vi "SubVI_RampingDrive_TeleOp.vi"(8 "error in (no error)":errorcluster, 10 "joystick Y Input":dbl) -> (0 "error out":errorcluster, 2 "joystick Y Output":dbl)   [LabVIEW 2017]
uses:
  <vilib>/Rock Robotics/WPI/Solenoid/WPI_SolenoidValue.ctl
  <vilib>/Rock Robotics/WPI/ThirdParty/Phoenix-LabVIEW/Motor Controller/Get/CTRE_Phoenix_MotorController_GetSelectedSensorData.vi
  <vilib>/Rock Robotics/WPI/Solenoid/WPI_SolenoidSetEnum.vi
panel:
  out "joystick Y Output 2":dbl
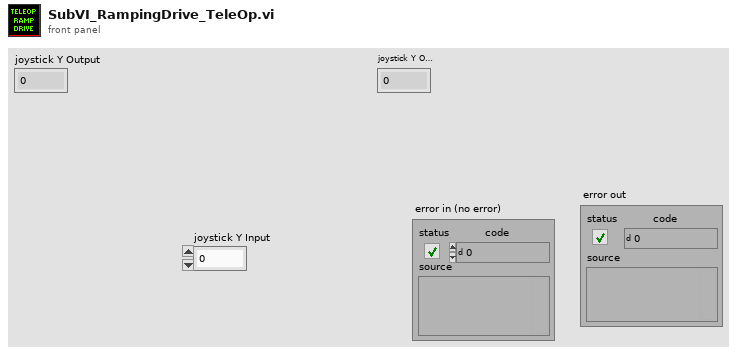
[diagram p1: front panel]
types:
  T1 = typedef "WPI_SolenoidValue.ctl" = enum16{"Off", "On", "Forward", "Reverse"}
  T2 = typedef "WPI_MotorControlDeviceRef.ctl" = cluster{"DeviceStatus":errorcluster, "Type":T3, "PWM":cluster{"PWM Channel":T4, "DeadBand":T5}, "CAN":cluster{"Device Number":u8, "SetOutput VI Ref":variant, "GetOutput VI Ref":variant, "Enable VI Ref":variant, "Disable VI Ref":variant, "Data":variant}, "Invert":bool, "DIO PWM":cluster{"PWM \"Enable\" Channel":T4, "DIOChannel":T6, "PWM Rate":dbl}}
  T3 = typedef "WPI_MotorControlType.ctl" = enum16{"PWM", "CAN", "DIO PWM"}
  T4 = typedef "FPGA_DIOPWMChannel.ctl" = enum8{"PWM 0", "PWM 1", "PWM 2", "PWM 3", "PWM 4", "PWM 5", "PWM 6", "PWM 7", "PWM 8", "PWM 9", "PWM MXP 0", "PWM MXP 1", "PWM MXP 2", "PWM MXP 3", "PWM MXP 4", "PWM MXP 5", "PWM MXP 6", "PWM MXP 7", "PWM MXP 8", "PWM MXP 9", "Invalid"}
  T5 = typedef "WPI_PWMDeadband.ctl" = cluster{"Name":string, "maxPositivePwm":i32, "minPositivePwm":i32, "centerPwm":i32, "maxNegativePwm":i32, "minNegativePwm":i32, "angularRange":u16}
  T6 = typedef "FPGA_DIOChannel.ctl" = enum8{"DIO 0", "DIO 1", "DIO 2", "DIO 3", "DIO 4", "DIO 5", "DIO 6", "DIO 7", "DIO 8", "DIO 9", "DIO MXP 0", "DIO MXP 1", "DIO MXP 2", "DIO MXP 3", "DIO MXP 4", "DIO MXP 5", "DIO MXP 6", "DIO MXP 7", "DIO MXP 8", "DIO MXP 9", "DIO MXP 10", "DIO MXP 11", "DIO MXP 12", "DIO MXP 13", "DIO MXP 14", "DIO MXP 15", "SPI Port CS1", "SPI Port CS2", "SPI Port CS3", "SPI Port MISO", "SPI Port MOSI", "Invalid"}
  T7 = typedef "WPI_SolenoidDevRef.ctl" = cluster{"DevStatus":errorcluster, "Pneumatics Control Module":u8, "Forward Solenoid Channel":T8, "Reverse Solenoid Channel":T8}
  T8 = typedef "WPI_SolenoidChannel.ctl" = enum8{"Solenoid 0", "Solenoid 1", "Solenoid 2", "Solenoid 3", "Solenoid 4", "Solenoid 5", "Solenoid 6", "Solenoid 7", "Invalid"}
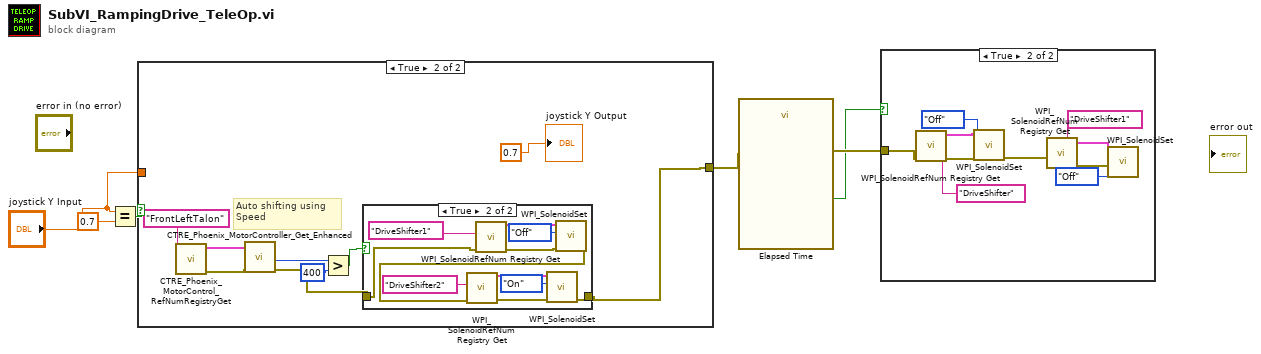
[diagram p0: block diagram]
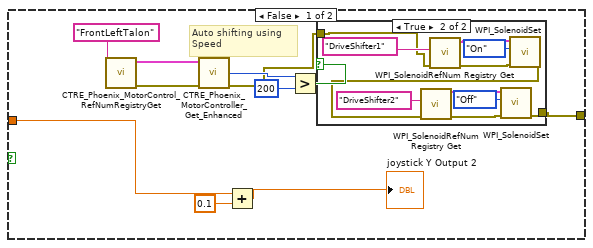
[diagram p3: hidden frame]
diagram:
  n1 = Equal?(x="joystick Y Input", y=0.7) -> (x = y?=w5:bool)
  n2 = case shown="True" w5 {
    tunnel: "joystick Y Input" -> [w17 _]
    tunnel: [w8 w30] -> w3
    frame False {
      # "Auto shifting using \nSpeed"
      n3 = call <vilib>:"CTRE_Phoenix_MotorControl_RefNumRegistryGet.vi"("refnum name"="FrontLeftTalon") -> ("error out"=w9:errorcluster, "PhoenixMotorControlDevRef"=w10:T2)  [unwired: 9 in]
      n4 = call-poly <vilib>:"CTRE_Phoenix_MotorController_Get_Enhanced.vi"("PhoenixMotorControlDevRef"=w10, "error in"=w9) -> ("Velocity (Raw Sensor Units per 100 ms)"=w14:i32, "error out"=w7:errorcluster)  [unwired: 10 in, 2 out]
      n5 = Add(x=w17, y=0.1) -> (x+y=→"joystick Y Output 2":dbl)
      n6 = Greater?(x=w14, y=200) -> (0:w12:bool)
      n7 = case shown="True" w12 {
        tunnel: [_ w19] -> w8
        tunnel: w7 -> [_ w18]
        frame False {
        }
        frame True {
          n8 = call <vilib>:"WPI_SolenoidRefNum Registry Get.vi"("error in (no error)"=w18, "refnum name"="DriveShifter1") -> ("error out"=w28:errorcluster, "SolenoidDevRef"=w23:T7)  [unwired: 8 in]
          n9 = call-poly <vilib>:"WPI_SolenoidSet.vi"("error in (no error)"=w28, "Value"=WPI_SolenoidValue."On", "SolenoidDevRef"=w23) -> ("error out"=w21:errorcluster)  [unwired: 7 in, 1 out]
          n10 = call <vilib>:"WPI_SolenoidRefNum Registry Get.vi"("error in (no error)"=w21, "refnum name"="DriveShifter2") -> ("error out"=w20:errorcluster, "SolenoidDevRef"=w22:T7)  [unwired: 8 in]
          n11 = call-poly <vilib>:"WPI_SolenoidSet.vi"("error in (no error)"=w20, "Value"=WPI_SolenoidValue."Off", "SolenoidDevRef"=w22) -> ("error out"=w19:errorcluster)  [unwired: 7 in, 1 out]
        }
      }
    }
    frame True {
      # "Auto shifting using \nSpeed"
      n12 = call <vilib>:"CTRE_Phoenix_MotorControl_RefNumRegistryGet.vi"("refnum name"="FrontLeftTalon") -> ("error out"=w31:errorcluster, "PhoenixMotorControlDevRef"=w32:T2)  [unwired: 9 in]
      n13 = call-poly <vilib>:"CTRE_Phoenix_MotorController_Get_Enhanced.vi"("PhoenixMotorControlDevRef"=w32, "error in"=w31) -> ("Velocity (Raw Sensor Units per 100 ms)"=w36:i32, "error out"=w29:errorcluster)  [unwired: 10 in, 2 out]
      n14 = Greater?(x=w36, y=400) -> (0:w34:bool)
      n15 = case shown="True" w34 {
        tunnel: [w38 w40] -> w30
        tunnel: w29 -> [w38 w39]
        frame False {
        }
        frame True {
          n16 = call <vilib>:"WPI_SolenoidRefNum Registry Get.vi"("error in (no error)"=w39, "refnum name"="DriveShifter1") -> ("error out"=w49:errorcluster, "SolenoidDevRef"=w44:T7)  [unwired: 8 in]
          n17 = call-poly <vilib>:"WPI_SolenoidSet.vi"("error in (no error)"=w49, "Value"=WPI_SolenoidValue."Off", "SolenoidDevRef"=w44) -> ("error out"=w41:errorcluster)  [unwired: 7 in, 1 out]
          n18 = call <vilib>:"WPI_SolenoidRefNum Registry Get.vi"("error in (no error)"=w41, "refnum name"="DriveShifter2") -> ("error out"=w43:errorcluster, "SolenoidDevRef"=w42:T7)  [unwired: 8 in]
          n19 = call-poly <vilib>:"WPI_SolenoidSet.vi"("error in (no error)"=w43, "Value"=WPI_SolenoidValue."On", "SolenoidDevRef"=w42) -> ("error out"=w40:errorcluster)  [unwired: 7 in, 1 out]
        }
      }
      "joystick Y Output" <- 0.7 ("joystick Output")
    }
  }
  n20 = call "Elapsed Time"("error in (no error)"=w3) -> ("Time has Elapsed"=w1:bool, "error out"=w2:errorcluster)  [unwired: 11 in, 6 out]
  n21 = case shown="True" w1 {
    tunnel: w2 -> [_ w53]
    frame False {
    }
    frame True {
      n22 = call <vilib>:"WPI_SolenoidRefNum Registry Get.vi"("error in (no error)"=w53, "refnum name"="DriveShifter") -> ("error out"=w52:errorcluster, "SolenoidDevRef"=w59:T7)  [unwired: 8 in]
      n23 = call-poly <vilib>:"WPI_SolenoidSet.vi"("error in (no error)"=w52, "Value"=WPI_SolenoidValue."Off", "SolenoidDevRef"=w59) -> ("error out"=w51:errorcluster)  [unwired: 7 in, 1 out]
      n24 = call <vilib>:"WPI_SolenoidRefNum Registry Get.vi"("error in (no error)"=w51, "refnum name"="DriveShifter1") -> ("error out"=w50:errorcluster, "SolenoidDevRef"=w56:T7)  [unwired: 8 in]
      n25 = call-poly <vilib>:"WPI_SolenoidSet.vi"("error in (no error)"=w50, "Value"=WPI_SolenoidValue."Off", "SolenoidDevRef"=w56) -> ()  [unwired: 7 in, 2 out]
    }
  }
